vi "Actor Core.vi"(8 "error in":errorcluster, 11 "Nested in":refnum<class "Products Picker.lvclass">) -> (0 "error out":errorcluster, 3 "Actor out":refnum<class "Actor.lvclass">)   [LabVIEW 2020, in "Products Picker.lvlib" / "Products Picker.lvclass"]
doc: "(<B>Filename</B>: Actor Framework.lvlib:Actor.lvclass:Actor Core.vi)\n\nReceives messages to the actor, reacts to them, and initiates any error handling that may shut the actor down.\n\nDescendant classes may override this VI to append parallel tasks for the actor to complete while it handles messages. Overrides use the Call Parent Method node."
uses:
  Products Picker.lvclass
  C:/Program Files (x86)/National Instruments/LabVIEW 2020/vi.lib/ActorFramework/Actor/Actor.lvclass
  <vilib>/ActorFramework/Actor/Actor.lvclass
  <vilib>/ActorFramework/Actor/Actor.lvclass/Actor.ctl
  <vilib>/ActorFramework/Message Enqueuer/Message Enqueuer.lvclass/Message Enqueuer.ctl
  Products Picker.lvclass/Products Picker.ctl
  Products Picker Messages/Product Selection Msg/Product Selection Msg.lvclass/Product Selection Msg.ctl
  <vilib>/ActorFramework/Message Enqueuer/Init from Existing Queue.vi
  <vilib>/ActorFramework/Message Enqueuer/Enqueue.vi
  <vilib>/ActorFramework/Stop Msg/Stop Msg.lvclass
  C:/Program Files (x86)/National Instruments/LabVIEW 2020/vi.lib/ActorFramework/Message/Message.lvclass
  Products Picker Messages/Product Selection Msg/Product Selection Msg.lvclass
  <vilib>/ActorFramework/Message Priority Queue/Priority Enqueue.vi
  <vilib>/ActorFramework/Message Enqueuer/Message Enqueuer.lvclass
panel:
  in  "Products":i32(listbox)
  out "Product Selected":string
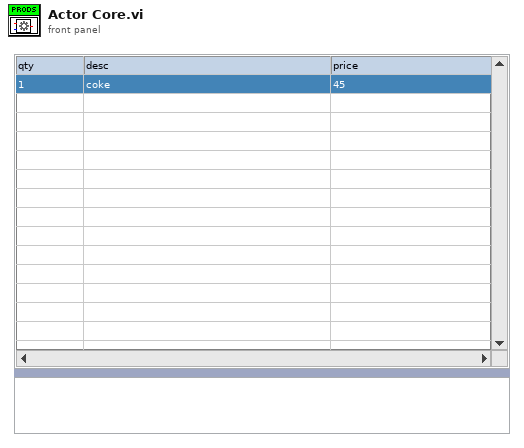
[diagram p1: front panel]
types:
  T1 = cluster{"Stop":refnum<user-event>, "Product Selected":refnum<user-event>}
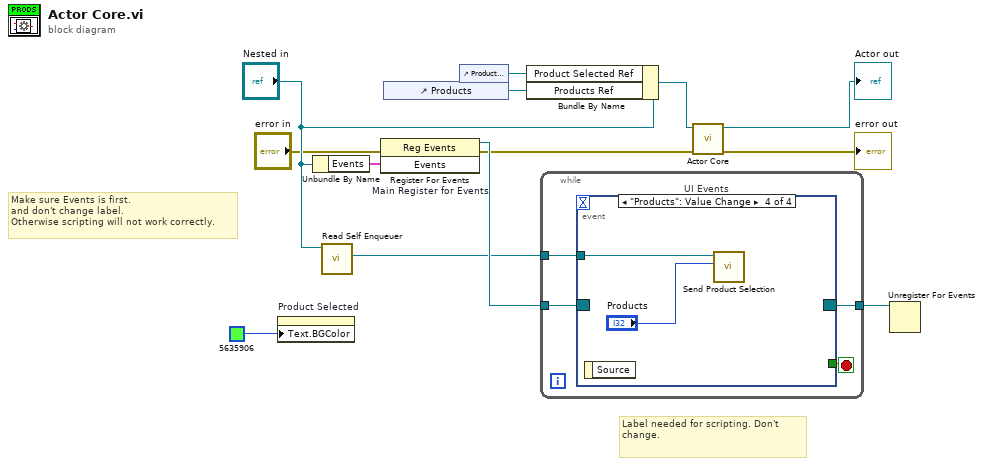
[diagram p0: block diagram]
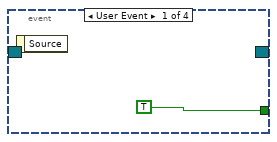
[diagram p2: hidden frame]
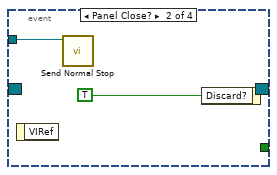
[diagram p3: hidden frame]
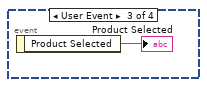
[diagram p4: hidden frame]
diagram:
  # "Label needed for scripting. Don't change."
  # "Make sure Events is first.\nand don't change label.\nOtherwise scripting will not work correctly."
  n1 = property on="Product Selected" class="Str"("Text.BGColor"=u32 5635906) -> ()  [unwired: 2 in, 2 out]
  n2 = Unbundle By Name("Nested in") -> ("Events"=w10:T1)
  n3 = call <vilib>:"Read Self Enqueuer.vi"("Actor"="Nested in") -> ("Self Enqueuer"=w7:refnum<class "Message Enqueuer.lvclass">)  [unwired: 10 in]
  n4 = register-events "Main Register for Events"(error in="error in", w10) -> (reference out=w11:refnum<event-registration>, error out=w5:errorcluster)  [unwired: 1 in]
  n5 = control-ref of="Products"() -> (w3:refnum<vi>)
  n6 = control-ref of="Product Selected"() -> (w1:refnum<vi>)
  n7 = Bundle By Name(cluster="Nested in", "Product Selected Ref"=w1, "Products Ref"=w3) -> (w4:refnum<class "Products Picker.lvclass">)
  n8 = while {
    tunnel: w11 -> [w17]
    tunnel: [w15] -> w9
    tunnel: w7 -> [w14]
    stop <- w16 stop-if-true
    n9 = event "UI Events" shown="[3] \"Products\": Value Change" {
      selector: w17 -> [_ _ _ _]
      dyn-events: [_ _ _ _] -> w15
      timeout: _ -> [_ _ _ _]
      tunnel: [TRUE _ _ _] -> w16
      tunnel: w14 -> [_ w19 _ w23]
      event User Event {
        n10 = event-data() -> ()  [unwired: 1 in, 1 out]
      }
      event Panel Close? {
        n11 = event-data() -> ()  [unwired: 1 in, 1 out]
        n12 = call <vilib>:"Send Normal Stop.vi"("Message Enqueuer"=w19) -> ()  [unwired: 10 in, 1 out]
        n13 = event-data("Discard?"=TRUE) -> ()  [unwired: 1 in, 1 out]
      }
      event User Event {
        n14 = event-data() -> ("Product Selected"=→"Product Selected":string)  [unwired: 1 in]
      }
      event "Products": Value Change {
        n15 = event-data() -> ()  [unwired: 1 in, 1 out]
        n16 = call "Send Product Selection.vi"("Products"="Products", "Message Enqueuer"=w23) -> ()  [unwired: 8 in, 2 out]
      }
    }
  }
  n17 = call-parent "Actor Core.vi"("error in"=w5, "Actor in"=w4) -> ("error out"=→"error out":errorcluster, "Actor out"=→"Actor out":refnum<class "Actor.lvclass">)  [unwired: 8 in]
  n18 = Unregister For Events(event registration refnum=w9) -> ()  [unwired: 1 in, 1 out]
